vi "call_c.vi"(11 "Extract dir":path) -> (0 "error out":errorcluster, 2 "standard error":string, 3 "standard output":string)   [LabVIEW 2023]
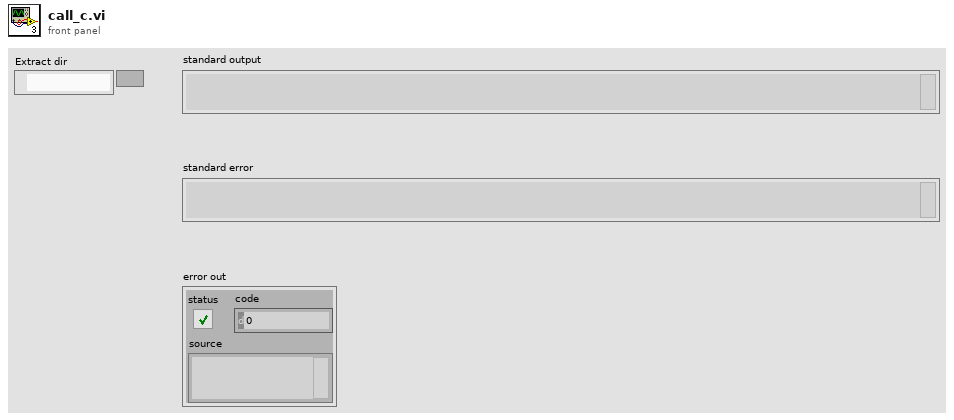
[diagram p1: front panel]
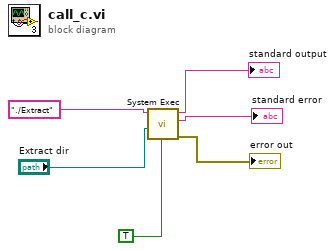
[diagram p0: block diagram]
diagram:
  n1 = call <vilib>:"System Exec.vi"("run minimized? (F)"=TRUE, "working directory"="Extract dir", "command line"="./Extract") -> ("error out"=→"error out":errorcluster, "standard error"=→"standard error":string, "standard output"=→"standard output":string)  [unwired: 5 in, 1 out]
